vi "Set_Tunnel_Speed.vi"(3 "Mode":T1, 5 "Tunnel Velocity m/s":dbl min=0.0 max=50.0 format="%.2f") -> (0 "Error String":string)   [LabVIEW 2012]
doc: "This is an example of using features of the VI Server as a client. It shows how you might browse from one or more applications that may be exporting data from one or more data stations. \n\nThe example shows how to query a server for its list of exported VIs, how to get references to the VIs, and how call them with the Call By Reference function."
uses:
  Sub VIs/ADAM Controls/Tunnel_speed_mode.ctl
  Anemometry/Anemometry Sub Vis/File/Setup_Filetype.ctl
  Sub VIs/ADAM Controls/Update_scan_value.ctl
  Anemometry/Anemometry Sub Vis/Controls/Global_mode.ctl
  Sub VIs/ADAM Controls/Ch_description_ADAM.ctl
  Sub VIs/ADAM Controls/Module_type_ADAM.ctl
  Sub VIs/ADAM Controls/Function_ADAM.ctl
  Sub VIs/ADAM Controls/Channel_State.ctl
  Sub VIs/ADAM Controls/Calib_type_ADAM.ctl
  Sub VIs/ADAM Controls/Address.ctl
  Anemometry/Anemometry Sub Vis/Globals/Preference_global.vi
  Anemometry/Anemometry Sub Vis/Globals/Trav_pos_global.vi
  <vilib>/Analysis/baseanly.llb/Mean (DBL).vi
  Anemometry/Anemometry Sub Vis/Globals/Constants_global.vi
  <vilib>/Analysis/NI_AALBase.lvlib
panel:
  in  "Set EnFlo Tun Speed":refnum<vi>
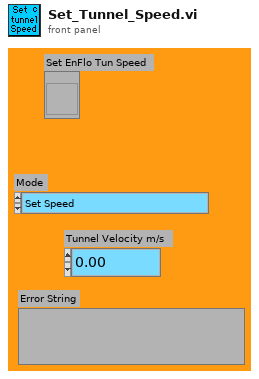
[diagram p1: front panel]
types:
  T1 = typedef "Tunnel_speed_mode.ctl" = enum16{"Set Speed", "Set Speed then wait", "Is tunnel speed allowable?"}
  T2 = typedef "Setup_Filetype.ctl" = enum16{"Measurement Setups", "Calibration Setups", "General", "Results File Plotter Setups", "Speed Calib Tweaks"}
  T3 = typedef "Channel_State.ctl" = enum16{"On", "Off", "Always On", "Always Off"}
  T4 = typedef "Calib_type_ADAM.ctl" = enum16{"Raw", "Bx + A", "Cx^2 + Bx + A", "Dx^3 + Cx^2 + Bx + A", "In Band", "Hi-Tec Q", "Hi-Tec M_dot", "Text"}
  T5 = typedef "Module_type_ADAM.ctl" = string
  T6 = typedef "Ch_description_ADAM.ctl" = cluster{"Ch Name":string, "Type":T5, "Function":T7, "Ch State":T3, "Calibration type":T4, "A":dbl, "B":dbl, "C":dbl, "D":dbl, "Comments":string, "Address":T8, "String":string, "Duty":u16}
  T7 = typedef "Function_ADAM.ctl" = enum16{"Analogue Input", "Digital Input", "Event counter", "Event rate", "Analogue Output", "Digital Output", "Relay Output"}
  T8 = typedef "Address.ctl" = cluster{"Main":i32, "Ch.":i32, "Sub":i32, "Port Name":string}
  T9 = typedef "Global_mode.ctl" = enum16{"Read Global", "Load Global From File", "Write Global to File"}
  T10 = typedef "Update_scan_value.ctl" = cluster{"Channel Name":string, "New Value":dbl}
  T11 = typedef "Server_Comms.ctl" = enum16{"Server Link Healthy", "Do Not Link To Server"}
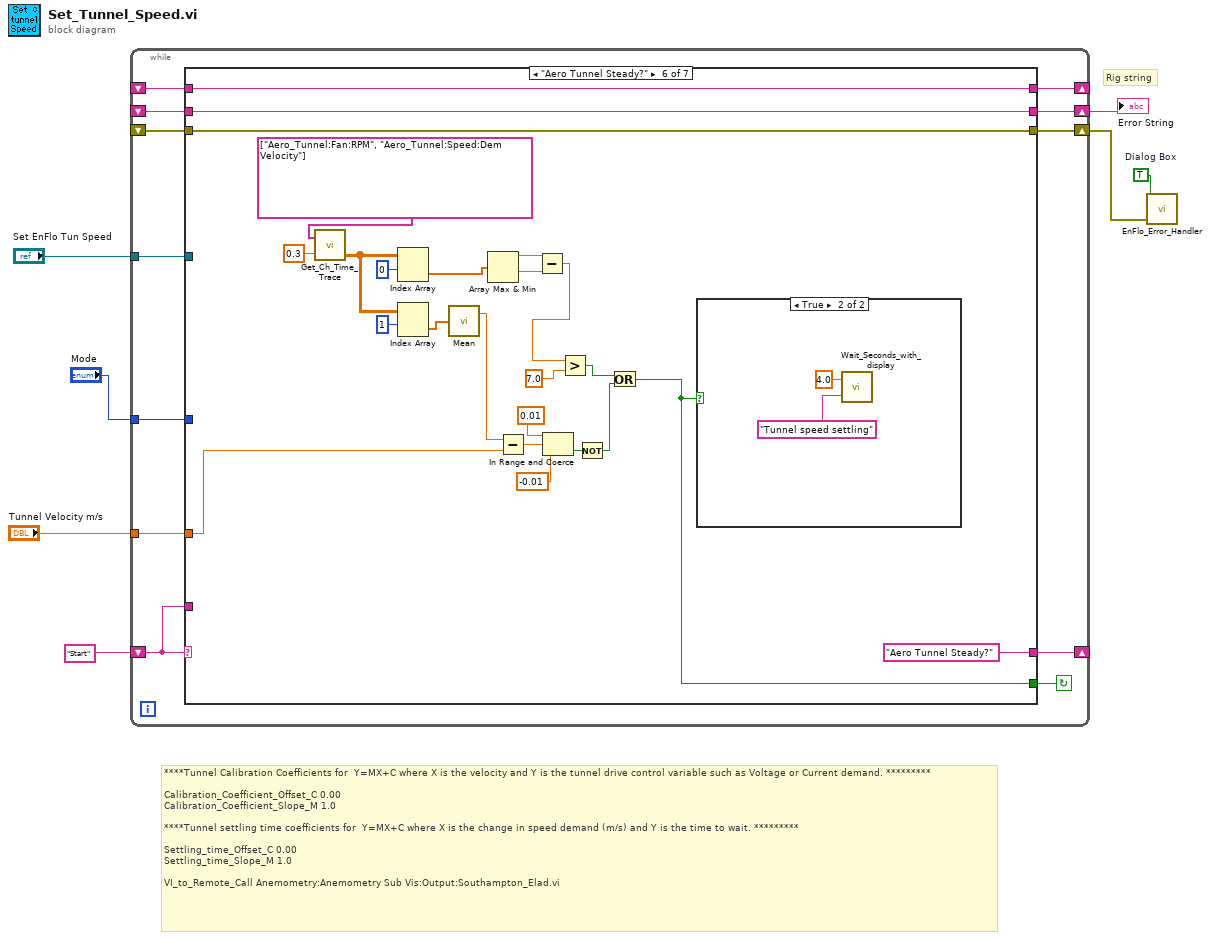
[diagram p0: block diagram]
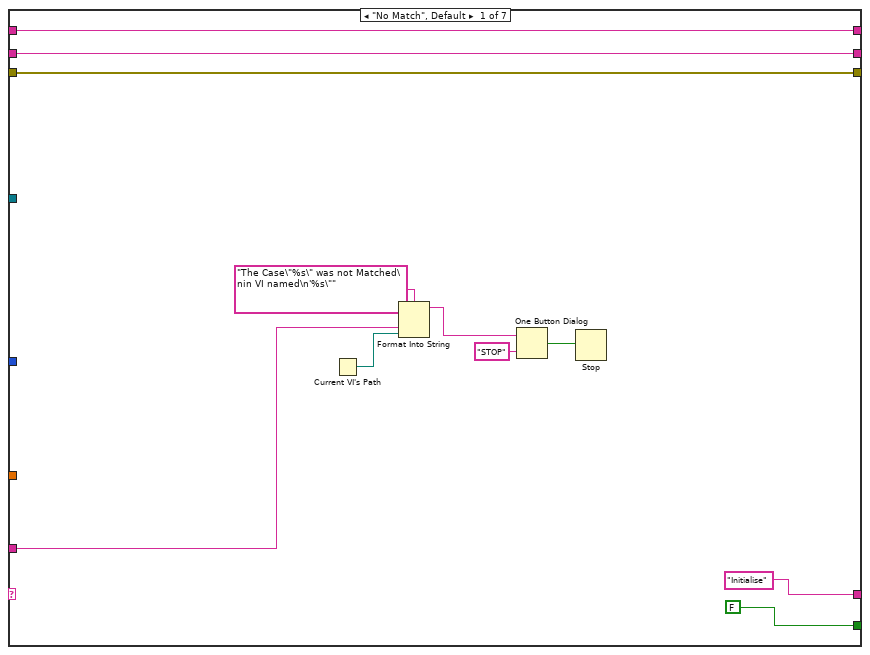
[diagram p2: hidden frame]
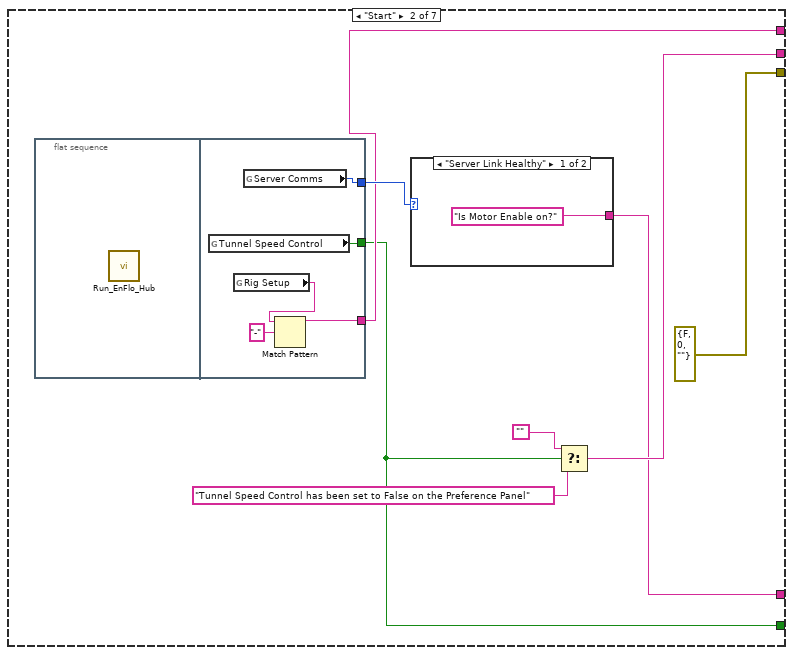
[diagram p3: hidden frame]
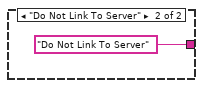
[diagram p4: hidden frame]
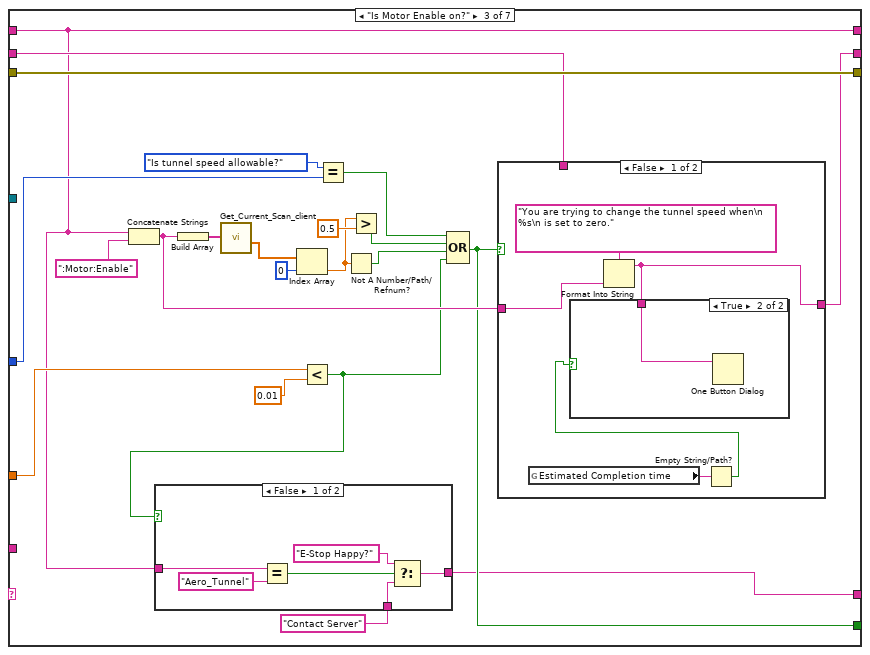
[diagram p5: hidden frame]
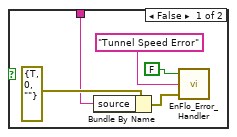
[diagram p7: hidden frame]
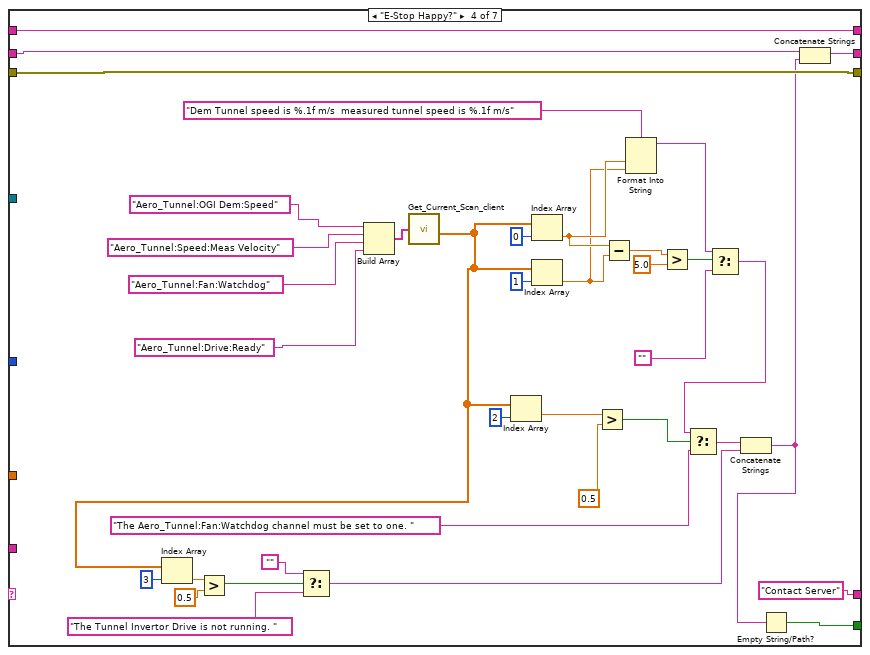
[diagram p9: hidden frame]
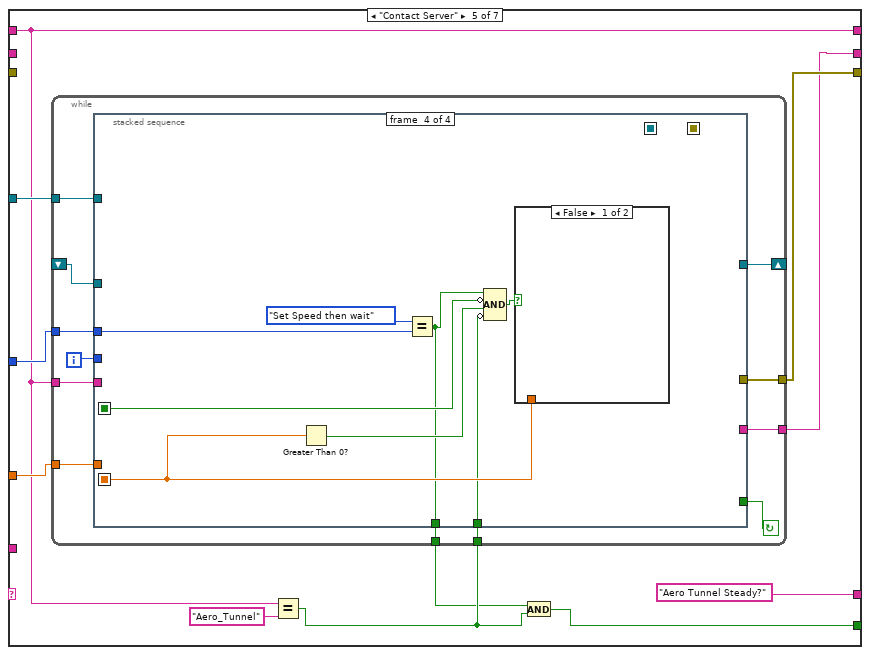
[diagram p10: hidden frame]
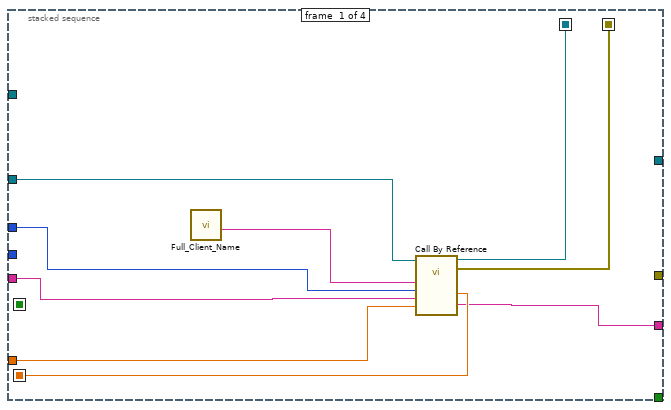
[diagram p11: hidden frame]
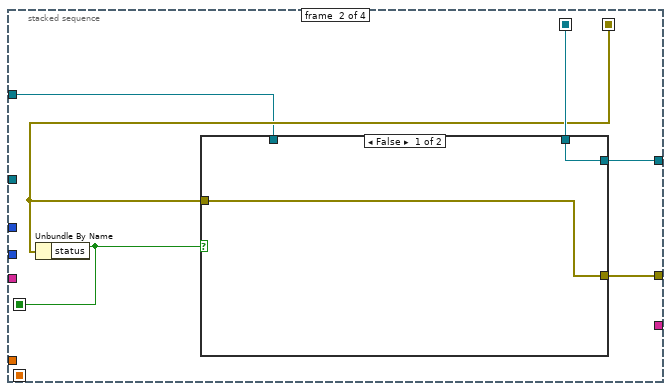
[diagram p12: hidden frame]
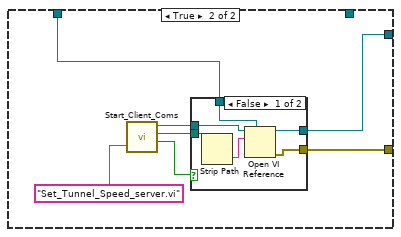
[diagram p13: hidden frame]
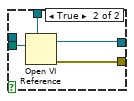
[diagram p14: hidden frame]
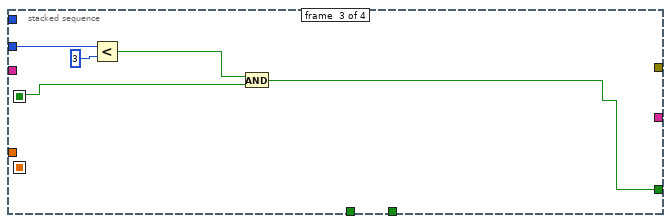
[diagram p15: hidden frame]
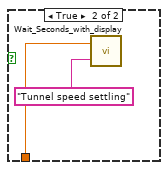
[diagram p16: hidden frame]
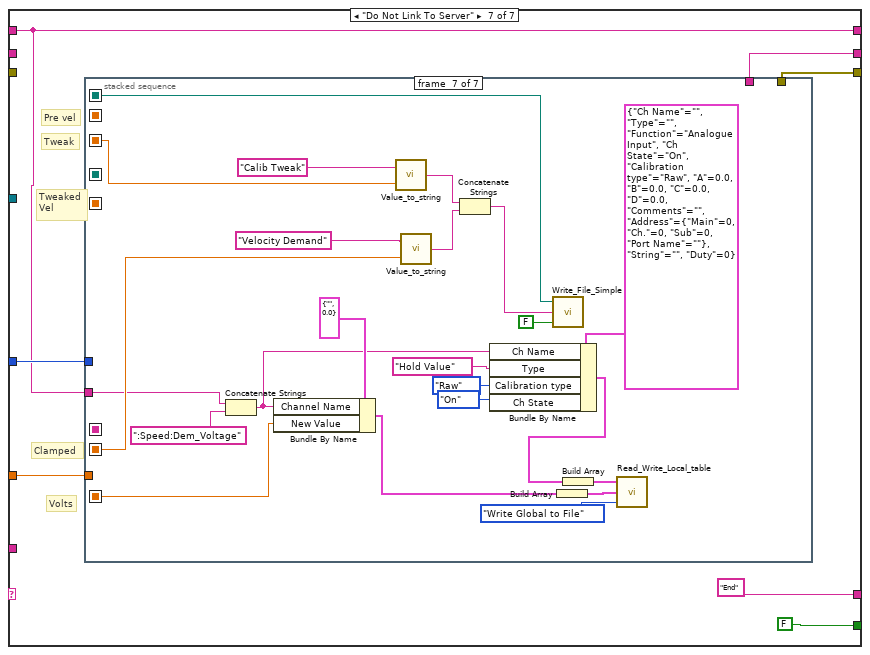
[diagram p18: hidden frame]
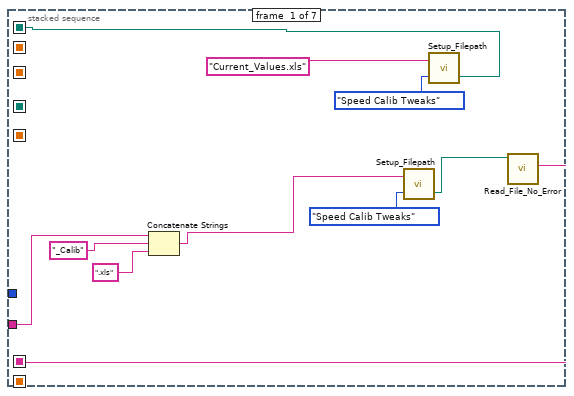
[diagram p19: hidden frame]
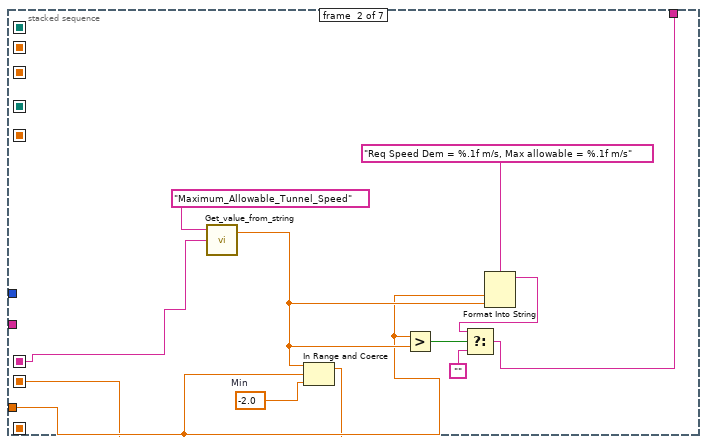
[diagram p20: hidden frame]
diagram:
  w7 = TRUE  # Dialog Box
  # "Rig string"
  # "****Tunnel Calibration Coefficients for  Y=MX+C where X is the velocity and Y is the tunnel drive control variable such as Voltage or Current demand. *********\n\nCalibration_Coefficient_Offset_C\t0.00\nCalibration_Coefficient_Slope_M\t1.0\n\n****Tunnel settling time coefficients for  Y=MX+C where X is the change in speed demand (m/s) and Y is the time to wait. *********\n\nSettling_time_Offset_C\t0.00\nSettling_time_Slope_M\t1.0\n\nVI_to_Remote_Call\tAnemometry:Anemometry Sub Vis:Output:Southampton_Elad.vi"
  n1 = while {
    shift-left: "Start" -> [w18]
    shift-right: [w19] -> _
    shift-right: [w17] -> w5
    shift-left: _ -> [w16]
    shift-right: [w15] -> w4
    shift-left: _ -> [w10]
    tunnel: "Mode" -> [w14]
    tunnel: "Tunnel Velocity m/s" -> [w13]
    shift-right: [w12] -> _
    shift-left: _ -> [w11]
    tunnel: "Set EnFlo Tun Speed" -> [w8]
    stop <- w9 continue-if-true
    n2 = case shown="\"Aero Tunnel Steady?\"" w18 {
      tunnel: [FALSE w35 w53 w100 w124 w201 FALSE] -> w9
      tunnel: ["Initialise" w31 w46 "Contact Server" ("f") "Aero Tunnel Steady?" ("f") "Aero Tunnel Steady?" ("f") "End"] -> w19
      tunnel: w18 -> [w25 _ _ _ _ _ _]
      tunnel: [w22 w33 w55 w114 w131 w217 w224] -> w17
      tunnel: w16 -> [w22 _ w54 w115 _ w217 _]
      tunnel: [w20 errorcluster {"status"=FALSE, "code"=0, "source"=""} ("error out") w57 w109 w132 w216 w223] -> w15
      tunnel: w14 -> [_ _ w51 _ w134 _ w226]
      tunnel: w13 -> [_ _ w58 _ w133 w208 w225]
      tunnel: [w21 w36 w49 w123 w128 w218 w222] -> w12
      tunnel: w11 -> [w21 _ w49 w123 w128 w218 w222]
      tunnel: w10 -> [w20 _ w57 w109 _ w216 _]
      tunnel: w8 -> [_ _ _ _ w130 _ _]
      frame "No Match", Default {
        n3 = Current VI's Path() -> (path=w24:path)
        n4 = Format Into String(format string="The Case\"%s\" was not Matched\nin VI named\n'%s\"" ("Format String"), w25, w24) -> (resulting string=w28:string)  [unwired: 2 in, 1 out]
        n5 = One Button Dialog(message=w28, button name ("OK")="STOP") -> (true=w26:bool)
        n6 = Stop(stop? (T)=w26) -> ()
      }
      frame "Start" {
        n7 = flat-sequence {
          tunnel: [w45] -> w38
          tunnel: [w44] -> w35
          tunnel: [w41] -> w36
          frame #0 {
            n8 = call "Run_EnFlo_Hub.vi"() -> ()  [unwired: 8 out]
          }
          frame #1 {
            n9 = global read "Preference_global.vi" "Tunnel Speed Control"() -> (w44:bool)
            n10 = global read "Preference_global.vi" "Rig Setup"() -> (w43:string)
            n11 = global read "Preference_global.vi" "Server Comms"() -> (w45:T11)
            n12 = Match Pattern(string=w43, regular expression="-") -> (before substring=w41:string)  [unwired: 4 out]
          }
        }
        n13 = case shown="\"Server Link Healthy\"" w38 {
          tunnel: ["Is Motor Enable on?" "Do Not Link To Server"] -> w31
          frame "Server Link Healthy" {
          }
          frame "Do Not Link To Server" {
          }
        }
        n14 = Select(t="", s=w35, f="Tunnel Speed Control has been set to False on the Preference Panel" ("Error String")) -> (s? t:f=w33:string)
      }
      frame "Is Motor Enable on?" {
        n15 = Concatenate Strings(w49, ":Motor:Enable" ("string")) -> (w56:string)
        n16 = Build Array(w56) -> (w60:string[])
        n17 = call "Get_Current_Scan_client.vi"("ADAM Ch Names"=w60) -> ("Numerical Values"=w61:dbl[])  [unwired: 3 out]
        n18 = Index Array(array=w61, index=0) -> (element=w63:dbl)
        n19 = Less?(x=w58, y=0.01) -> (x < y?=w48:bool)
        n20 = case shown="False" w48 {
          tunnel: w49 -> [w72 _]
          tunnel: [w70 w74] -> w46
          tunnel: "Contact Server" ("f") -> [w68 w74]
          frame False {
            n21 = Equal?(x=w72, y="Aero_Tunnel") -> (x = y?=w71:bool)
            n22 = Select(t="E-Stop Happy?" ("f"), s=w71, f=w68) -> (s? t:f=w70:string)
          }
          frame True {
          }
        }
        n23 = Equal?(x=Tunnel_speed_mode."Is tunnel speed allowable?" ("Mode"), y=w51) -> (x = y?=w50:bool)
        n24 = Not A Number/Path/Refnum?(number/path/refnum=w63) -> (NaN/Path/Refnum?=w65:bool)
        n25 = Greater?(x=w63, y=0.5) -> (0:w66:bool)
        n26 = Compound Arithmetic op=OR(w50, w66, w65, w48) -> (w53:bool)
        n27 = case shown="False" w53 {
          tunnel: w56 -> [w78 _]
          tunnel: [w75 w86] -> w55
          tunnel: w54 -> [_ w86]
          frame False {
            n28 = global read "Trav_pos_global.vi" "Estimated Completion time"() -> (w77:string)
            n29 = Format Into String(format string="You are trying to change the tunnel speed when\n %s\n is set to zero.", w78) -> (resulting string=w75:string)  [unwired: 2 in, 1 out]
            n30 = Empty String/Path?(string/path=w77) -> (empty?=w76:bool)
            n31 = case shown="True" w76 {
              tunnel: w75 -> [w81 w85]
              frame False {
                n32 = Bundle By Name(cluster=errorcluster {"status"=TRUE, "code"=0, "source"=""} ("error in (no error)"), "source"=w81) -> (w82:errorcluster)
                n33 = call "EnFlo_Error_Handler.vi"("error in (no error)"=w82, "Error Type"="Tunnel Speed Error", "Dialog Box (T)"=FALSE) -> ()  [unwired: 3 out]
              }
              frame True {
                n34 = One Button Dialog(message=w85) -> ()  [unwired: 2 out]
              }
            }
          }
          frame True {
          }
        }
      }
      frame "E-Stop Happy?" {
        n35 = Build Array("Aero_Tunnel:OGI Dem:Speed", "Aero_Tunnel:Speed:Meas Velocity", "Aero_Tunnel:Fan:Watchdog", "Aero_Tunnel:Drive:Ready") -> (w120:string[])
        n36 = call "Get_Current_Scan_client.vi"("ADAM Ch Names"=w120) -> ("Numerical Values"=w97:dbl[])  [unwired: 1 in, 2 out]
        n37 = Index Array(array=w97, index=3) -> (element=w96:dbl)
        n38 = Greater?(x=w96, y=0.5) -> (0:w94:bool)
        n39 = Select(t="", s=w94, f="The Tunnel Invertor Drive is not running. ") -> (s? t:f=w90:string)
        n40 = Index Array(array=w97, index=2) -> (element=w104:dbl)
        n41 = Index Array(array=w97, index=0) -> (element=w113:dbl)
        n42 = Index Array(array=w97, index=1) -> (element=w112:dbl)
        n43 = Greater?(x=w104, y=0.5) -> (0:w87:bool)
        n44 = Subtract(x=w113, y=w112) -> (x-y=w117:dbl)
        n45 = Format Into String(format string="Dem Tunnel speed is %.1f m/s  measured tunnel speed is %.1f m/s", w113, w112) -> (resulting string=w110:string)  [unwired: 2 in, 1 out]
        n46 = Greater?(x=w117, y=5.0) -> (0:w107:bool)
        n47 = Select(t=w110, s=w107, f="") -> (s? t:f=w102:string)
        n48 = Select(t=w102, s=w87, f="The Aero_Tunnel:Fan:Watchdog channel must be set to one. ") -> (s? t:f=w91:string)
        n49 = Concatenate Strings(w91, w90) -> (w89:string)
        n50 = Empty String/Path?(string/path=w89) -> (empty?=w100:bool)
        n51 = Concatenate Strings(w115, w89) -> (w114:string)
      }
      frame "Contact Server" {
        n52 = Equal?(x=w128, y="Aero_Tunnel") -> (x = y?=w126:bool)
        n53 = while {
          tunnel: w134 -> [w141]
          tunnel: w133 -> [w142]
          tunnel: [w143] -> w132
          shift-left: _ -> [w138]
          shift-right: [w146] -> _
          tunnel: [w140] -> w131
          tunnel: w128 -> [w139]
          tunnel: w130 -> [w137]
          tunnel: w126 -> [w136]
          tunnel: [w135] -> w125
          i -> [w145]
          stop <- w144 continue-if-true
          n54 = stacked-sequence {
            seq-local: [w154 _ _ _] -> [_ w160 _ _]
            seq-local: [w153 _ _ _] -> [_ w158 _ _]
            seq-local: [_ w159 _ _] -> [_ _ w182 w189]
            seq-local: [w150 _ _ _] -> [_ _ _ w192]
            tunnel: w138 -> [w155 _ _ _]
            tunnel: [_ w161 _ _] -> w146
            tunnel: w145 -> [_ _ w183 _]
            tunnel: [_ _ w181 _] -> w144
            tunnel: [_ w157 _ _] -> w143
            tunnel: w142 -> [w151 _ _ _]
            tunnel: w141 -> [w147 _ _ w193]
            tunnel: [w149 _ _ _] -> w140
            tunnel: w139 -> [w148 _ _ _]
            tunnel: w137 -> [_ w156 _ _]
            tunnel: w136 -> [_ _ _ w187]
            tunnel: [_ _ _ w186] -> w135
            frame #0 {
              n55 = call "Full_Client_Name.vi"() -> ("Client Name"=w152:string)
              n56 = call-by-ref "?"(reference=w155, "Tunnel Velocity m/s"=w151, "Rig Name"=w148, "Mode"=w147, "Client Name"=w152) -> (reference out=w154:refnum<vi>, error out=w153:errorcluster, "Error String"=w149:string, "Settling Time (s)"=w150:dbl)  [unwired: 1 in, 1 out]
            }
            frame #1 {
              n57 = Unbundle By Name(w158) -> ("status"=w159:bool)
              n58 = case shown="False" w159 {
                tunnel: [w162 w166] -> w161
                tunnel: w160 -> [w162 _]
                tunnel: [w163 w165] -> w157
                tunnel: w158 -> [w163 _]
                tunnel: w156 -> [_ w164]
                frame False {
                }
                frame True {
                  n59 = call "Start_Client_Coms.vi"("VI name to run on server"="Set_Tunnel_Speed_server.vi") -> ("LabVIEW application reference"=w168:refnum<vi>, "Checked VI name"=w169:path, "Local Call"=w167:bool)  [unwired: 1 in, 1 out]
                  n60 = case shown="False" w167 {
                    tunnel: [w175 w180] -> w166
                    tunnel: w164 -> [w173 w179]
                    tunnel: w169 -> [w172 w178]
                    tunnel: w168 -> [w171 _]
                    tunnel: [w174 w177] -> w165
                    frame False {
                      n61 = Strip Path(path=w172) -> (name=w176:string)  [unwired: 1 out]
                      n62 = Open VI Reference(type specifier VI Refnum (for type only)=w173, application reference (local)=w171, vi path=w176) -> (vi reference=w175:refnum<vi>, error out=w174:errorcluster)  [unwired: 1 in, 2 out]
                    }
                    frame True {
                      n63 = Open VI Reference(type specifier VI Refnum (for type only)=w179, vi path=w178) -> (vi reference=w180:refnum<vi>, error out=w177:errorcluster)  [unwired: 1 in, 3 out]
                    }
                  }
                }
              }
            }
            frame #2 {
              n64 = Less?(x=w183, y=3) -> (x < y?=w185:bool)
              n65 = And(x=w185, y=w182) -> (x .and. y?=w181:bool)
            }
            frame #3 {
              n66 = Greater Than 0?(x=w192) -> (x > 0?=w188:bool)
              n67 = Equal?(x=Tunnel_speed_mode."Set Speed then wait" ("Mode"), y=w193) -> (x = y?=w186:bool)
              n68 = Compound Arithmetic op=AND(w186, invert w189, w188, invert w187) -> (w190:bool)
              n69 = case shown="False" w190 {
                tunnel: w192 -> [_ w194]
                frame False {
                }
                frame True {
                  n70 = call "Wait_Seconds_with_display.vi"("Message"="Tunnel speed settling", "Seconds to wait"=w194) -> ()  [unwired: 2 out]
                }
              }
            }
          }
        }
        n71 = And(x=w125, y=w126) -> (x .and. y?=w124:bool)
      }
      frame "Aero Tunnel Steady?" {
        n72 = call "Get_Ch_Time_Trace.vi"("Desired Ch Names"=string[] ["Aero_Tunnel:Fan:RPM", "Aero_Tunnel:Speed:Dem Velocity"] ("ADAM Ch Names"), "History Length (mins)"=0.3) -> ("Output array"=w211:dbl[][])  [unwired: 2 out]
        n73 = Index Array(array=w211, index (row)=0) -> (element=w207:dbl[])  [unwired: 1 in]
        n74 = Index Array(array=w211, index (row)=1) -> (element=w210:dbl[])  [unwired: 1 in]
        n75 = call-poly <vilib>:"Mean.vi"("X"=w210) -> ("mean"=w209:dbl)  [unwired: 1 out]
        n76 = Array Max & Min(array=w207) -> (max value=w206:dbl, min value=w205:dbl)  [unwired: 2 out]
        n77 = Subtract(x=w209, y=w208) -> (x-y=w198:dbl)
        n78 = Subtract(x=w206, y=w205) -> (x-y=w204:dbl)
        n79 = In Range and Coerce(upper limit=0.01, x=w198, lower limit=-0.01) -> (In Range?=w197:bool)  [unwired: 1 out]
        n80 = Greater?(x=w204, y=7.0) -> (0:w202:bool)
        n81 = Not(x=w197) -> (.not. x?=w196:bool)
        n82 = Or(x=w202, y=w196) -> (x .or. y?=w201:bool)
        n83 = case shown="True" w201 {
          frame False {
          }
          frame True {
            n84 = call "Wait_Seconds_with_display.vi"("Message"="Tunnel speed settling", "Seconds to wait"=4.0) -> ()  [unwired: 2 out]
          }
        }
      }
      frame "Do Not Link To Server" {
        # "Clamped"
        # "Pre vel"
        # "Tweak"
        # "Tweaked\nVel"
        # "Volts"
        n85 = stacked-sequence {
          seq-local: [w235 _ _ _ _ _ _] -> [_ w249 w255 w263 w279 w338 _]
          seq-local: [_ _ w250 _ _ _ _] -> [_ _ _ _ w283 _ _]
          seq-local: [_ _ _ w259 _ _ _] -> [_ _ _ _ w278 _ w351]
          seq-local: [_ _ _ w262 _ _ _] -> [_ _ _ _ w281 w333 _]
          seq-local: [_ _ _ _ w280 _ _] -> [_ _ _ _ _ w332 _]
          seq-local: [_ _ _ w264 _ _ _] -> [_ _ _ _ _ _ w357]
          seq-local: [w232 _ _ _ _ _ _] -> [_ _ _ _ _ _ w359]
          seq-local: [_ w240 _ _ _ _ _] -> [_ _ _ w257 _ _ w356]
          tunnel: w225 -> [_ w241 _ _ _ _ _]
          tunnel: w222 -> [w236 _ _ w272 _ _ w353]
          tunnel: w226 -> [_ _ _ _ w282 w327 _]
          tunnel: [_ w239 _ _ _ _ _] -> w224
          tunnel: [_ _ _ _ w277 _ _] -> w223
          frame #0 {
            n86 = Concatenate Strings(w236, "_Calib" ("Substring"), ".xls" ("string")) -> (w230:string)
            n87 = call "Setup_Filepath.vi"("Setup File Type"=Setup_Filetype."Speed Calib Tweaks", "Filename in"=w230) -> ("Filename Out"=w229:path)  [unwired: 1 out]
            n88 = call "Setup_Filepath.vi"("Setup File Type"=Setup_Filetype."Speed Calib Tweaks", "Filename in"="Current_Values.xls" ("name or relative path")) -> ("Filename Out"=w232:path)  [unwired: 1 out]
            n89 = call "Read_File_No_Error.vi"("Filename"=w229) -> ("string"=w235:string)  [unwired: 2 in, 7 out]
          }
          frame #1 {
            w243 = -2.0  # Min
            n90 = call "Get_value_from_string.vi"("Input string"=w249, "Variable name"="Maximum_Allowable_Tunnel_Speed") -> ("Value"=w242:dbl)  [unwired: 1 in, 1 out]
            n91 = In Range and Coerce(upper limit=w242, x=w241, lower limit=w243) -> (coerced(x)=w240:dbl)  [unwired: 1 out]
            n92 = Greater?(x=w241, y=w242) -> (0:w244:bool)
            n93 = Format Into String(format string="Req Speed Dem = %.1f m/s, Max allowable = %.1f m/s", w241, w242) -> (resulting string=w246:string)  [unwired: 2 in, 1 out]
            n94 = Select(t=w246, s=w244, f="") -> (s? t:f=w239:string)
          }
          frame #2 {
            n95 = call "Get_Characters_from_string.vi"("Input string"=w255, "Variable name"="VI_to_Remote_Call") -> ("Value"=w253:string)  [unwired: 1 in, 1 out]
            n96 = global read "Constants_global.vi" "EnFlo SW Folder"() -> (w251:path)
            n97 = call "String_to_Pathname.vi"("Input String"=w253) -> ("path"=w254:path)
            n98 = Path to Array of Strings(0:w254) -> (2:w252:string[])  [unwired: 1 out]
            n99 = call "Build_Pathname.vi"("PathElements"=w252, "PathnameIn"=w251) -> ("AppendedPath"=w250:path)
          }
          frame #3 {
            w270 = FALSE  # Tunnel Heated?
            n100 = local write "Tunnel Velocity m/s"(w257) -> ()
            n101 = call "Add_to_speed_calib_file.vi"("Desired Velocity"=w257, "Tunnel Heated?"=w270, "Rig Name"=w272, "Mode"=enum16{"Add Row", "Get Error Value"}."Get Error Value") -> ("Tweaked Demand"=w262:dbl, "Calib Tweak %"=w264:dbl)  [unwired: 2 in]
            n102 = Less?(x=w262, y=0.01) -> (x < y?=w260:bool)
            n103 = call "Get_value_from_string.vi"("Input string"=w263, "Variable name"="Calibration_Coefficient_Offset_C") -> ("Value"=w265:dbl)  [unwired: 1 in, 1 out]
            n104 = call "Get_value_from_string.vi"("Input string"=w263, "Variable name"="Calibration_Coefficient_Slope_M") -> ("Value"=w267:dbl)  [unwired: 1 in, 1 out]
            n105 = Multiply(x=w267, y=w262) -> (x*y=w266:dbl)
            n106 = Add(x=w265, y=w266) -> (x+y=w258:dbl)
            n107 = case shown="False" w260 {
              tunnel: w263 -> [_ w275]
              tunnel: [w273 w274] -> w259
              tunnel: w258 -> [w273 _]
              frame False {
              }
              frame True {
                n108 = call "Get_value_from_string.vi"("Input string"=w275, "Variable name"="Zero_Velocity_Output_Voltage") -> ("Value"=w274:dbl)  [unwired: 1 in, 1 out]
              }
            }
          }
          frame #4 {
            n109 = while {
              tunnel: w283 -> [w293]
              tunnel: w282 -> [w292]
              tunnel: w281 -> [w291]
              tunnel: [w290] -> w280
              shift-right: [w288] -> _
              shift-left: _ -> [w287]
              tunnel: [w286] -> w277
              tunnel: w279 -> [w285]
              tunnel: w278 -> [w284]
              stop <- TRUE stop-if-true
              n110 = case shown="\"Set Speed then wait\", Default" w292 {
                tunnel: w293 -> [_ w313]
                tunnel: w291 -> [_ w300]
                tunnel: [w295 w302] -> w290
                tunnel: [w295 w300] -> w288
                tunnel: w287 -> [w295 w301]
                tunnel: [errorcluster {"status"=FALSE, "code"=0, "source"=""} ("error out") w296] -> w286
                tunnel: w285 -> [_ _]
                tunnel: w284 -> [_ w299]
                frame "Is tunnel speed allowable?" {
                }
                frame "Set Speed then wait", Default {
                  n111 = Open VI Reference(type specifier VI Refnum (for type only)=refnum<vi> refnum, vi path=w313) -> (vi reference=w311:refnum<vi>, error out=w310:errorcluster)  [unwired: 1 in, 3 out]
                  n112 = property class="VI Interface Type 0"(reference=w311, error in=w310) -> (reference out=w308:refnum<vi>, error out=w309:errorcluster, "Front Panel.Open"=w307:bool)
                  n113 = case shown="False" w307 {
                    tunnel: w309 -> [w318 w321]
                    tunnel: w308 -> [w317 w322]
                    tunnel: [w316 w322] -> w306
                    tunnel: [w315 w321] -> w305
                    tunnel: [0.0 ("Tweaked Demand") w320] -> w302
                    tunnel: w301 -> [_ w320]
                    frame False {
                      n114 = property class="VI Interface Type 0"(reference=w317, error in=w318, "Front Panel.Open"=TRUE ("Front Panel Window:Open")) -> (reference out=w316:refnum<vi>, error out=w315:errorcluster)
                    }
                    frame True {
                    }
                  }
                  n115 = call-by-ref "?"(reference=w306, error in=w305, "Demand"=w299) -> (reference out=w303:refnum<vi>, error out=w304:errorcluster, "error out"=w297:errorcluster)
                  n116 = Close Reference(reference=w303, error in (no error)=w304) -> (error out=w298:errorcluster)
                  n117 = Select(t=w298, s=w298, f=w297) -> (s? t:f=w296:errorcluster)
                }
              }
            }
          }
          frame #5 {
            n118 = Subtract(x=w332, y=w333) -> (x-y=w331:dbl)
            n119 = Absolute Value(x=w331) -> (abs(x)=w325:dbl)
            n120 = call "Get_value_from_string.vi"("Input string"=w338, "Variable name"="Settling_time_Offset_C") -> ("Value"=w334:dbl)  [unwired: 1 in, 1 out]
            n121 = call "Get_value_from_string.vi"("Input string"=w338, "Variable name"="Settling_time_Slope_M") -> ("Value"=w336:dbl)  [unwired: 1 in, 1 out]
            n122 = Multiply(x=w336, y=w325) -> (x*y=w335:dbl)
            n123 = Add(x=w334, y=w335) -> (x+y=w326:dbl)
            n124 = Greater?(x=w325, y=0.05) -> (0:w323:bool)
            n125 = Equal?(x=Tunnel_speed_mode."Set Speed then wait" ("Mode"), y=w327) -> (x = y?=w329:bool)
            n126 = Compound Arithmetic op=AND(w323, w329) -> (w328:bool)
            n127 = case shown="False" w328 {
              tunnel: w326 -> [_ w340]
              frame False {
              }
              frame True {
                n128 = call "Wait_Seconds_with_display.vi"("Message"="Tunnel speed settling", "Seconds to wait"=w340) -> ()  [unwired: 2 out]
              }
            }
          }
          frame #6 {
            n129 = Concatenate Strings(w353, ":Speed:Dem_Voltage" ("string")) -> (w348:string)
            n130 = Bundle By Name(cluster=T10 {"Channel Name"="", "New Value"=0.0} ("Update Scan Value Cluster"), "Channel Name"=w348, "New Value"=w351) -> (w354:T10)
            n131 = call "Value_to_string.vi"("Value"=w357, "Label for value"="Calib Tweak") -> ("Output string"=w362:string)  [unwired: 1 in]
            n132 = call "Value_to_string.vi"("Value"=w356, "Label for value"="Velocity Demand") -> ("Output string"=w361:string)  [unwired: 1 in]
            n133 = Concatenate Strings(w362, w361) -> (w360:string)
            n134 = Bundle By Name(cluster=T6 {"Ch Name"="", "Type"="", "Function"=enum."Analogue Input", "Ch State"=enum."On", "Calibration type"=enum."Raw", "A"=0.0, "B"=0.0, "C"=0.0, "D"=0.0, "Comments"="", "Address"={"Main"=0, "Ch."=0, "Sub"=0, "Port Name"=""}, "String"="", "Duty"=0} ("Ch Discription"), "Ch Name"=w348, "Type"=T5 "Hold Value", "Calibration type"=Calib_type_ADAM."Raw", "Ch State"=Channel_State."On") -> (w342:T6)
            n135 = call "Write_File_Simple.vi"("append to file? (new file:F)"=FALSE, "character string"=w360, "file path"=w359) -> ()  [unwired: 2 out]
            n136 = Build Array(w354) -> (w344:T10[])
            n137 = Build Array(w342) -> (w343:T6[])
            n138 = call "Read_Write_Local_table.vi"("Mode"=Global_mode."Write Global to File", "Ch Values in"=w344, "Channels Descriptions In"=w343) -> ()  [unwired: 3 out]
          }
        }
      }
    }
  }
  "Error String" <- w5
  n139 = call "EnFlo_Error_Handler.vi"("error in (no error)"=w4, "Dialog Box (T)"=w7) -> ()  [unwired: 1 in, 3 out]
